vi "Enum.vi"() -> ()   [LabVIEW 2022 SP3]
panel:
  out "Numeric 4":dbl
  out "Numeric 3":dbl
  in  "Numeric 2":dbl
  in  "Numeric":dbl
  in  "Enum":enum16{"PROCESS 1", "PROCESS 2", "PROCESS 3"}(ring)
  in  "Ring":u16(ring) items=["PROCESS 1", "PROCESS 2", "PROCESS 3"]
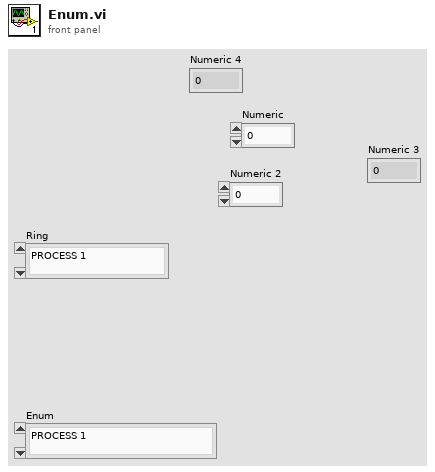
[diagram p1: front panel]
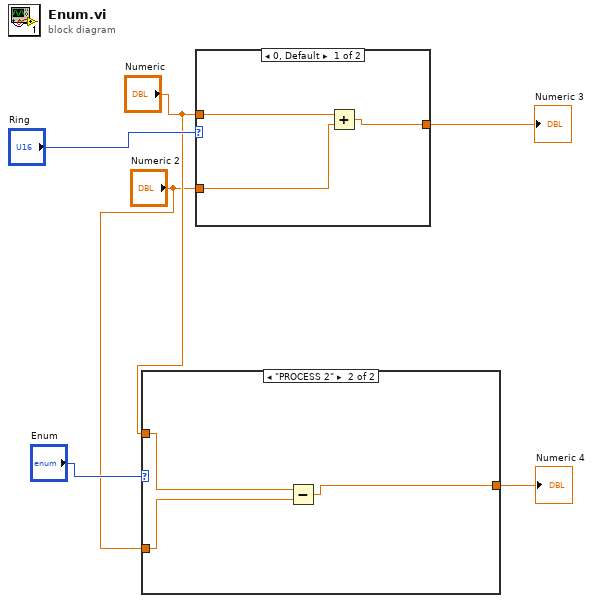
[diagram p0: block diagram]
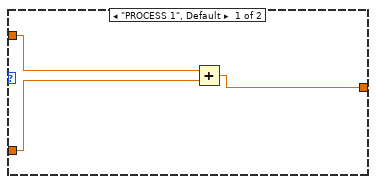
[diagram p2: hidden frame]
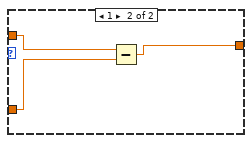
[diagram p3: hidden frame]
diagram:
  n1 = case shown="\"PROCESS 2\"" "Enum" {
    tunnel: "Numeric" -> [w8 w12]
    tunnel: "Numeric 2" -> [w7 w11]
    tunnel: [w9 w10] -> w1
    frame "PROCESS 1", Default {
      n2 = Add(x=w8, y=w7) -> (x+y=w9:dbl)
    }
    frame "PROCESS 2" {
      n3 = Subtract(x=w12, y=w11) -> (x-y=w10:dbl)
    }
  }
  "Numeric 4" <- w1
  n4 = case shown="0, Default" "Ring" {
    tunnel: "Numeric" -> [w15 w18]
    tunnel: "Numeric 2" -> [w14 w17]
    tunnel: [w13 w16] -> w5
    frame 0, Default {
      n5 = Add(x=w15, y=w14) -> (x+y=w13:dbl)
    }
    frame 1 {
      n6 = Subtract(x=w18, y=w17) -> (x-y=w16:dbl)
    }
  }
  "Numeric 3" <- w5
